vi "IonHeatingEnable.vi"(0 "Strings in":string[](array[string])=["C:\\CuspControl\\GPIB and Network\\Cusp\\Dummyfile.txt", "6723"], 1 "Dubs in":dbl[](array[numeric])=[0.011]) -> ()   [LabVIEW 2018]
uses:
  <vilib>/DAQmx/write.llb/DAQmx Write (Analog DBL 1Chan 1Samp).vi
  <vilib>/DAQmx/create/channels.llb/DAQmx Create Channel (AO-Voltage-Basic).vi
  <vilib>/DAQmx/miscellaneous.llb/DAQmx Fill In Error Info.vi
panel:
  in  "ON":bool
  in  "subvi":bool=TRUE
  out "error out":errorcluster
  in  "AO2 name":string="6723"
  in  "relay ao line":string="/ao3"
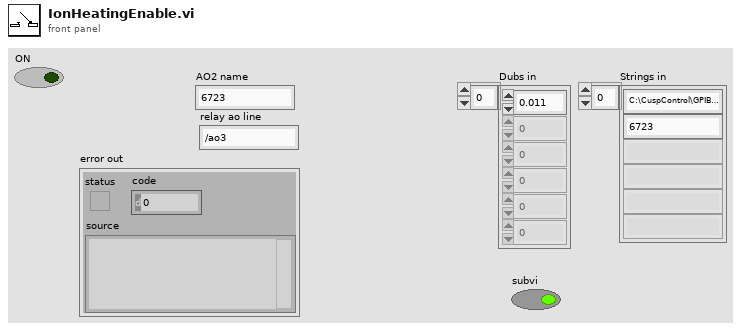
[diagram p1: front panel]
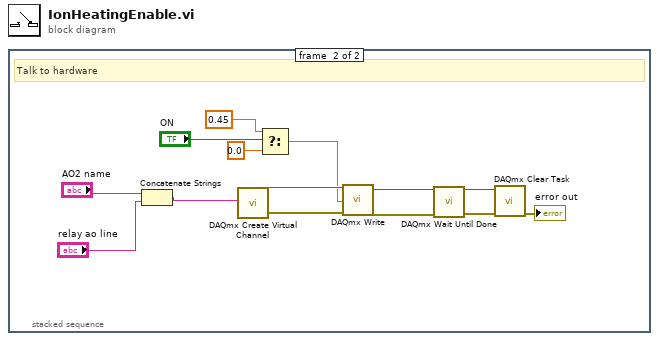
[diagram p0: block diagram]
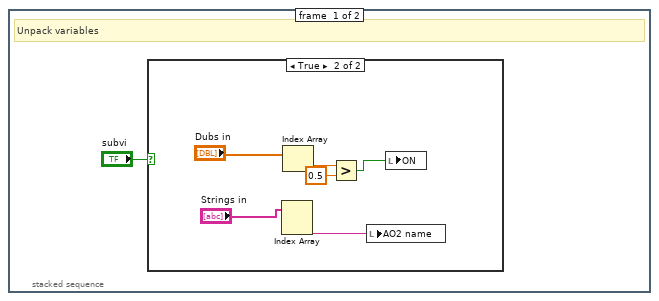
[diagram p2: hidden frame]
diagram:
  n1 = stacked-sequence {
    frame #0 {
      # "Unpack variables"
      n2 = case shown="True" "subvi" {
        frame False {
        }
        frame True {
          n3 = Index Array(array="Strings in") -> (element #2=w5:string)  [unwired: 2 in, 1 out]
          n4 = Index Array(array="Dubs in") -> (element=w4:dbl)  [unwired: 1 in]
          n5 = Greater?(x=w4, y=0.5) -> (0:w2:bool)
          n6 = local write "AO2 name"(w5) -> ()
          n7 = local write "ON"(w2) -> ()
        }
      }
    }
    frame #1 {
      # "Talk to hardware"
      n8 = Concatenate Strings("AO2 name", "relay ao line") -> (w15:string)
      n9 = call-poly <vilib>:"DAQmx Create Virtual Channel.vi"("physical channels"=w15) -> ("task out"=w21:refnum<k21>, "error out"=w20:errorcluster)  [unwired: 13 in]
      n10 = Select(t=0.45 ("ON voltage"), s="ON", f=0.0) -> (s? t:f=w10:dbl)
      n11 = call-poly <vilib>:"DAQmx Write.vi"("task/channels in"=w21, "data"=w10, "error in"=w20) -> ("task out"=w17:refnum<k21>, "error out"=w16:errorcluster)  [unwired: 10 in, 1 out]
      n12 = call <vilib>:"DAQmx Wait Until Done.vi"("task/channels in"=w17, "error in"=w16) -> ("task out"=w19:refnum<k21>, "error out"=w18:errorcluster)  [unwired: 12 in]
      n13 = call <vilib>:"DAQmx Clear Task.vi"("task in"=w19, "error in"=w18) -> ("error out"=→"error out":errorcluster)  [unwired: 13 in]
    }
  }
